vi "RSZVB Recall Limit Line With Options.vi"(4 "S-Parameter":string, 5 "Type (1: Upper)":i32(ring)=1 items=["Off", "Upper", "Lower"], 6 "Y Offset (0.0)":dbl format="%^.3e", 7 "X Offset (0.0)":dbl format="%^.3e", 8 "error in (no error)":errorcluster {"code" format="%.0x"}, 9 "File Name (Trc1.limit)":string="Trc1.limit", 10 "Trace Name (Trc1)":string="Trc1", 11 "VISA session":refnum<visa-resource-name>) -> (0 "error out":errorcluster {"code" format="%.0x"}, 3 "dup VISA session":refnum<visa-resource-name>)   [LabVIEW 2011]
doc: "This VI loads a limit line definition from a specified file and assigns it to a trace with a specified name. Limit lines are created using the CALCulte<Ch/Tr>:LIMit... commands.\n\nRemote-control command(s):\nMMEMory:LOAD:LIMit '<trc_name>','<file_name>'[,'<param_name>', <x_offset>, <y_offset>, <type>]"
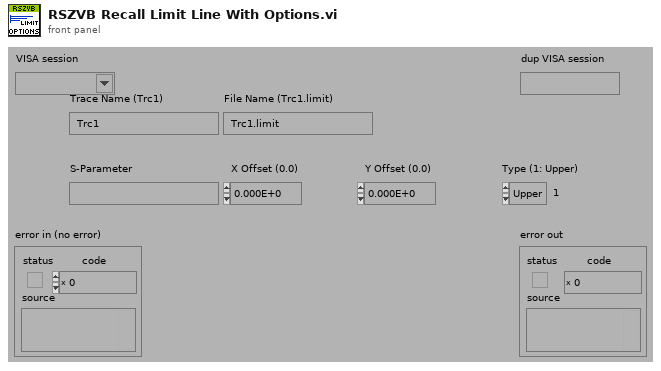
[diagram p1: front panel]
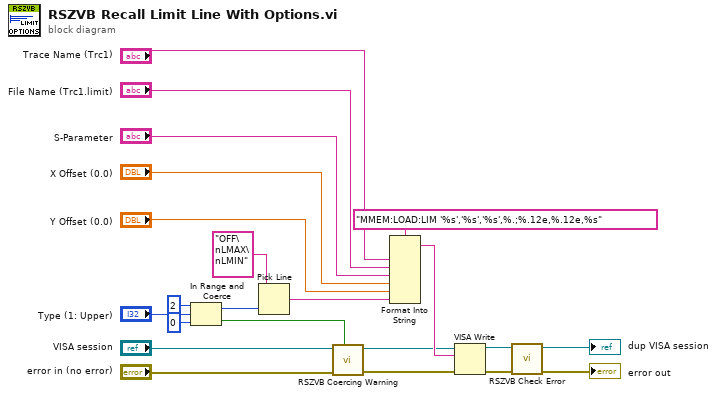
[diagram p0: block diagram]
diagram:
  n1 = In Range and Coerce(upper limit=2, x="Type (1: Upper)", lower limit=0) -> (coerced(x)=w6:i32, In Range?=w5:bool)
  n2 = Pick Line(multi-line string="OFF\nLMAX\nLMIN", line index=w6) -> (output string=w15:string)  [unwired: 1 in]
  n3 = call "RSZVB Coercing Warning.vi"("In Range?"=w5, "error in (no error)"="error in (no error)", "VISA session"="VISA session") -> ("error out"=w3:errorcluster, "dup VISA session"=w4:refnum<visa-resource-name>)  [unwired: 7 in]
  n4 = Format Into String(format string="MMEM:LOAD:LIM '%s','%s','%s',%.;%.12e,%.12e,%s", "Trace Name (Trc1)", "File Name (Trc1.limit)", "S-Parameter", "X Offset (0.0)", "Y Offset (0.0)", w15) -> (resulting string=w19:string)  [unwired: 2 in, 1 out]
  n5 = VISA Write(VISA resource name=w4, write buffer=w19, error in (no error)=w3) -> (VISA resource name out=w21:refnum<visa-resource-name>, error out=w22:errorcluster)  [unwired: 1 out]
  n6 = call "RSZVB Check Error.vi"("error in (no error)"=w22, "VISA session"=w21) -> ("error out"=→"error out":errorcluster, "dup VISA session"=→"dup VISA session":refnum<visa-resource-name>)  [unwired: 8 in]
